vi "Find Interface.vi"(8 "error in (no error)":errorcluster, 10 "Resource":refnum<visa-resource-name>, 11 "F4T in":refnum<class "F4T.lvclass">) -> (0 "error out":errorcluster, 1 "InterfaceType":i32(ring)=2 items=["Usb", "Serial", "Ethernet", "Unconnected"], 2 "Resource out":refnum<visa-resource-name>, 3 "F4T out":refnum<class "F4T.lvclass">)   [LabVIEW 2018, in "F4T.lvlib" / "F4T.lvclass"]
uses:
  F4T.lvclass
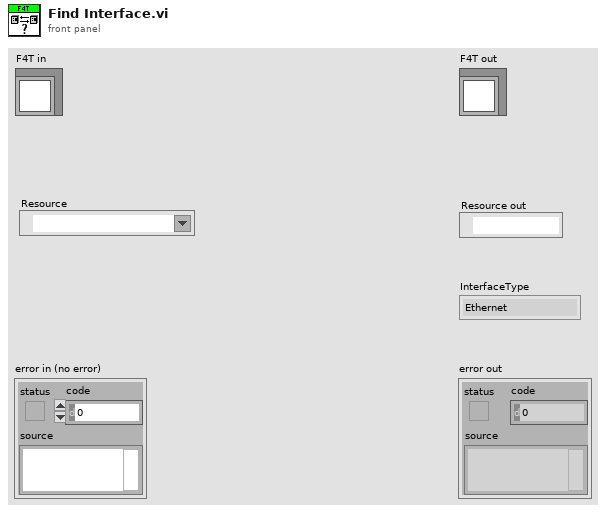
[diagram p1: front panel]
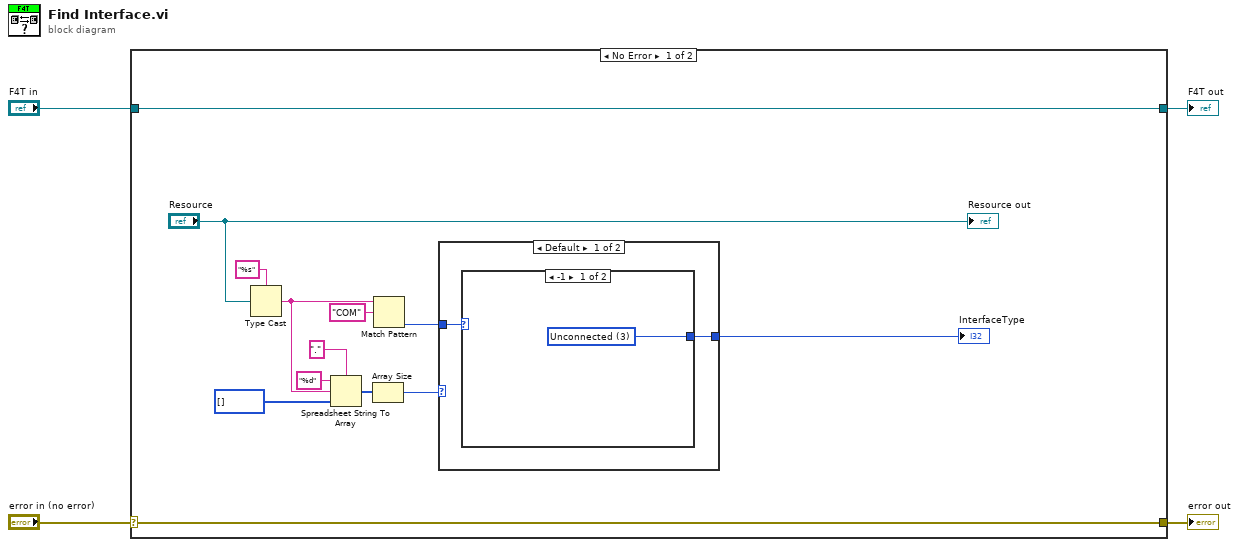
[diagram p0: block diagram]
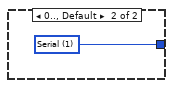
[diagram p2: hidden frame]
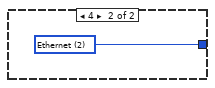
[diagram p3: hidden frame]
diagram:
  n1 = case shown="No Error" "error in (no error)" {
    selector: "error in (no error)" -> [w16 w24]
    tunnel: [w16 w24] -> w3
    tunnel: [w17 w23] -> w1
    tunnel: "F4T in" -> [w17 w23]
    frame No Error {
      n2 = Type Cast(type="%s", x="Resource") -> (*(type *) &x=w11:string)
      n3 = Spreadsheet String To Array(delimiter (Tab)=".", format string="%d", spreadsheet string=w11, array type (2D Dbl)=u8[] []) -> (array=w8:u8[])
      n4 = Array Size(array=w8) -> (size(s)=w7:i32)
      n5 = Match Pattern(string=w11, regular expression="COM") -> (offset past match=w5:i32)  [unwired: 1 in, 3 out]
      n6 = case shown="Default" w7 {
        tunnel: [w18 w22] -> w6
        tunnel: w5 -> [w19 _]
        frame Default {
          n7 = case shown="-1" w19 {
            tunnel: [w20 w21] -> w18
            frame -1 {
              w20 = 3 items=["Usb", "Serial", "Ethernet", "Unconnected"] ("InterfaceType")
            }
            frame 0.., Default {
              w21 = 1 items=["Usb", "Serial", "Ethernet", "Unconnected"] ("InterfaceType")
            }
          }
        }
        frame 4 {
          w22 = 2 items=["Usb", "Serial", "Ethernet", "Unconnected"] ("InterfaceType")
        }
      }
      "InterfaceType" <- w6
      "Resource out" <- "Resource"
    }
    frame Error {
    }
  }
  "error out" <- w3
  "F4T out" <- w1
